vi "DISP_WIND_TRAC_DEL.vi"(0 "VISA IN":refnum<visa-resource-name>, 1 "Trace":i32=1, 5 "error in":errorcluster, 7 "Window":i32=1) -> (14 "VISA Out":refnum<visa-resource-name>, 19 "error out":errorcluster)   [LabVIEW 2018, in "PNA-X.lvlib"]
doc: "DISPlay:WINDow<wnum>:TRACe<tnum>:DELete \n(Write-only) Deletes the specified trace from the specified window. The measurement parameter \nassociated with the trace is not deleted. \nParameters \n<wnum> Any existing window number. If unspecified, value is set to 1. \n<tnum> The number of the trace to be deleted; if unspecified, value is set to 1 \nExamples DISP:WIND:TRAC:DEL \ndisplay:window2:trace2:delete \nQuery Syntax Not applicable \nDefault NA"
uses:
  PNA-X.lvlib
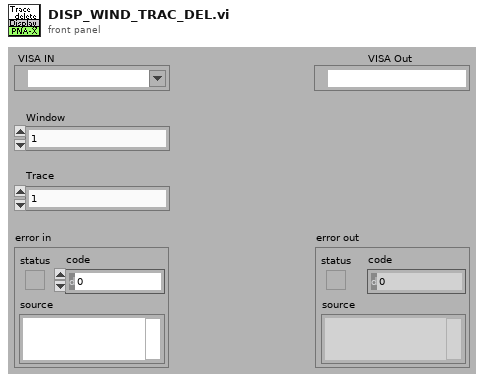
[diagram p1: front panel]
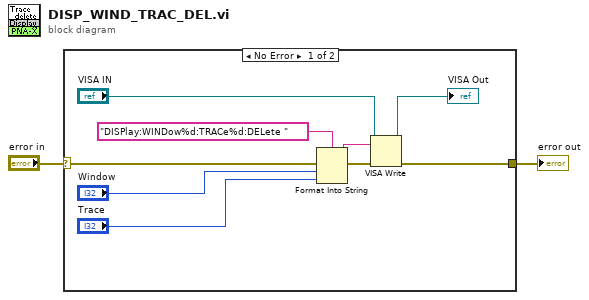
[diagram p0: block diagram]
diagram:
  n1 = case shown="No Error" "error in" {
    selector: "error in" -> [w11 w12]
    tunnel: [w6 w12] -> w1
    frame No Error {
      n2 = Format Into String(format string="DISPlay:WINDow%d:TRACe%d:DELete " ("Cmdline"), error in=w11, "Window", "Trace") -> (resulting string=w9:string, error out=w10:errorcluster)  [unwired: 1 in]
      n3 = VISA Write(VISA resource name="VISA IN", write buffer=w9, error in (no error)=w10) -> (VISA resource name out=→"VISA Out":refnum<visa-resource-name>, error out=w6:errorcluster)  [unwired: 1 out]
    }
    frame Error {
    }
  }
  "error out" <- w1
